vi "Read Black Start Status.vi"(11 "Black Start Status Msg in":refnum<class "Black Start Status Msg.lvclass">) -> (0 "Status":T1, 1 "error":string, 2 "Sequence":string, 3 "Black Start Status Msg out":refnum<class "Black Start Status Msg.lvclass">)   [LabVIEW 2015, in "SCADA Core.lvlib" / "Black Start Status Msg.lvclass"]
uses:
  Black Start Status Msg.lvclass
  Black Start Status.ctl
  Black Start Status Msg.lvclass/Black Start Status Msg.ctl
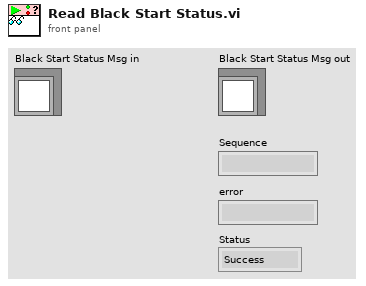
[diagram p1: front panel]
types:
  T1 = typedef "SCADA Core.lvlib/Black Start Status Msg.lvclass/Black Start Status.ctl" = enum16{"Success", "Failure"}
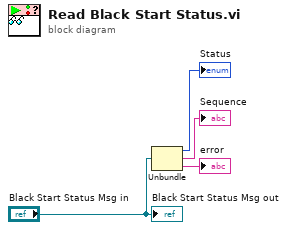
[diagram p0: block diagram]
diagram:
  n1 = Unbundle("Black Start Status Msg in") -> (→"Status":T1, →"Sequence":string, →"error":string)
  "Black Start Status Msg out" <- "Black Start Status Msg in"
